vi "Host3.vi"() -> ()   [LabVIEW 2025]
uses:
  <vilib>/Analysis/baseanly.llb/Real Dot Product.vi
  <vilib>/Analysis/baseanly.llb/Real A x B.vi
  <vilib>/Analysis/Matrix/Numeric/Conversions/Matrix To Array - RM.vi
  <vilib>/Utility/error.llb/Error Cluster From Error Code.vi
  <vilib>/rvi/errors/niLvFpgaAdjustHostInterfaceError.vi
  <vilib>/FPGAPlugInAG/Dynamic/niLvFpga_Run_Dynamic.vi
  <vilib>/FPGAPlugInAG/Dynamic/niLvFpga_Close_Dynamic.vi
  <vilib>/rvi/interface/nirviOpenFPGA/nirviOpenFPGA.xnode
  <vilib>/rvi/interface/nirviMethod/nirviMethod.xnode
  <vilib>/rvi/interface/nirviCloseFPGA/nirviCloseFPGA.xnode
  <vilib>/FPGAPlugInAG/Dynamic/niLvFpga_WriteFifo_Dynamic.vi
  <vilib>/rvi/errors/niLvFpgaMergeErrorWithErrorCode.vi
  <vilib>/Analysis/NI_AALBase.lvlib
  <vilib>/Analysis/Matrix/NI_Matrix.lvlib
  <vilib>/FPGAPlugInAG/Dynamic/niLvFpga_ReadFifo_Dynamic.vi
  FPGA Bitfiles/dotplot9033_FPGATarget_Target_CwM8WDNFVFM.lvbitx
  Target.vi
  <vilib>/FPGAPlugInAG/cRIO-9033/niLvFpga_Open_cRIO-9033.vi
  <vilib>/rvi/interface/common/dynamic/niFpgaDynamicAddResources.vi
panel:
  out "FIFO C Output":fxp<+/-,32,16>[](array[numeric])
  out "FIFO A Input":fxp<+/-,32,16>[](array[numeric])
  out "FIFO B Input":fxp<+/-,32,16>[](array[numeric])
  out "X * Y":fxp<+/-,64,32>
  out "elements in B":i32
  out "elements in A":i32
  out "sum of error":dbl
  out "C - FPGA code":fxp<+/-,32,16>[][](array[numeric])
  out "elements in C":i32
  out "C - Real":dbl[][](array[numeric])
  out "B":fxp<+/-,32,16>[][](array[numeric])
  out "A":fxp<+/-,32,16>[][](array[numeric])
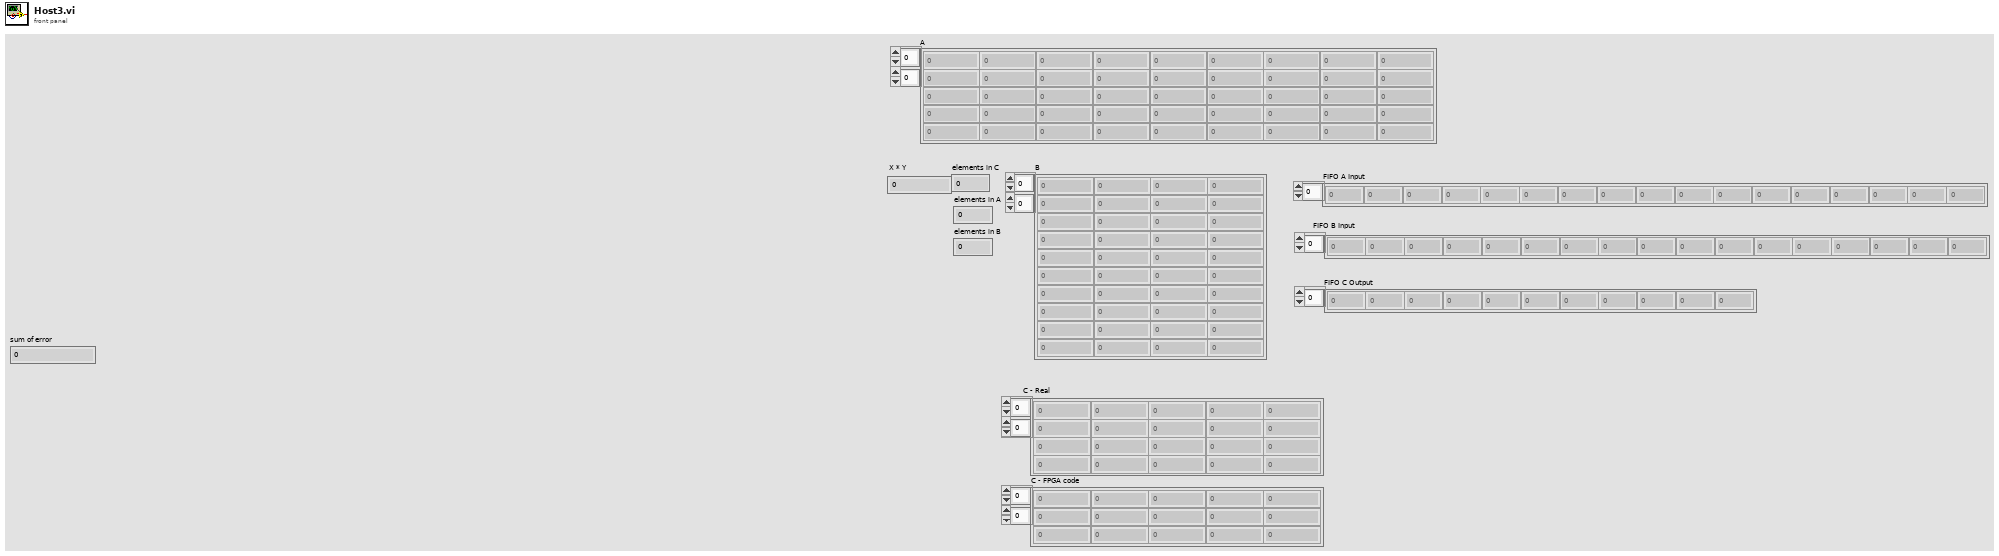
[diagram p1: front panel]
types:
  T1 = typedef "NI_Matrix.lvlib/RealMatrix.ctl" = dbl[][]
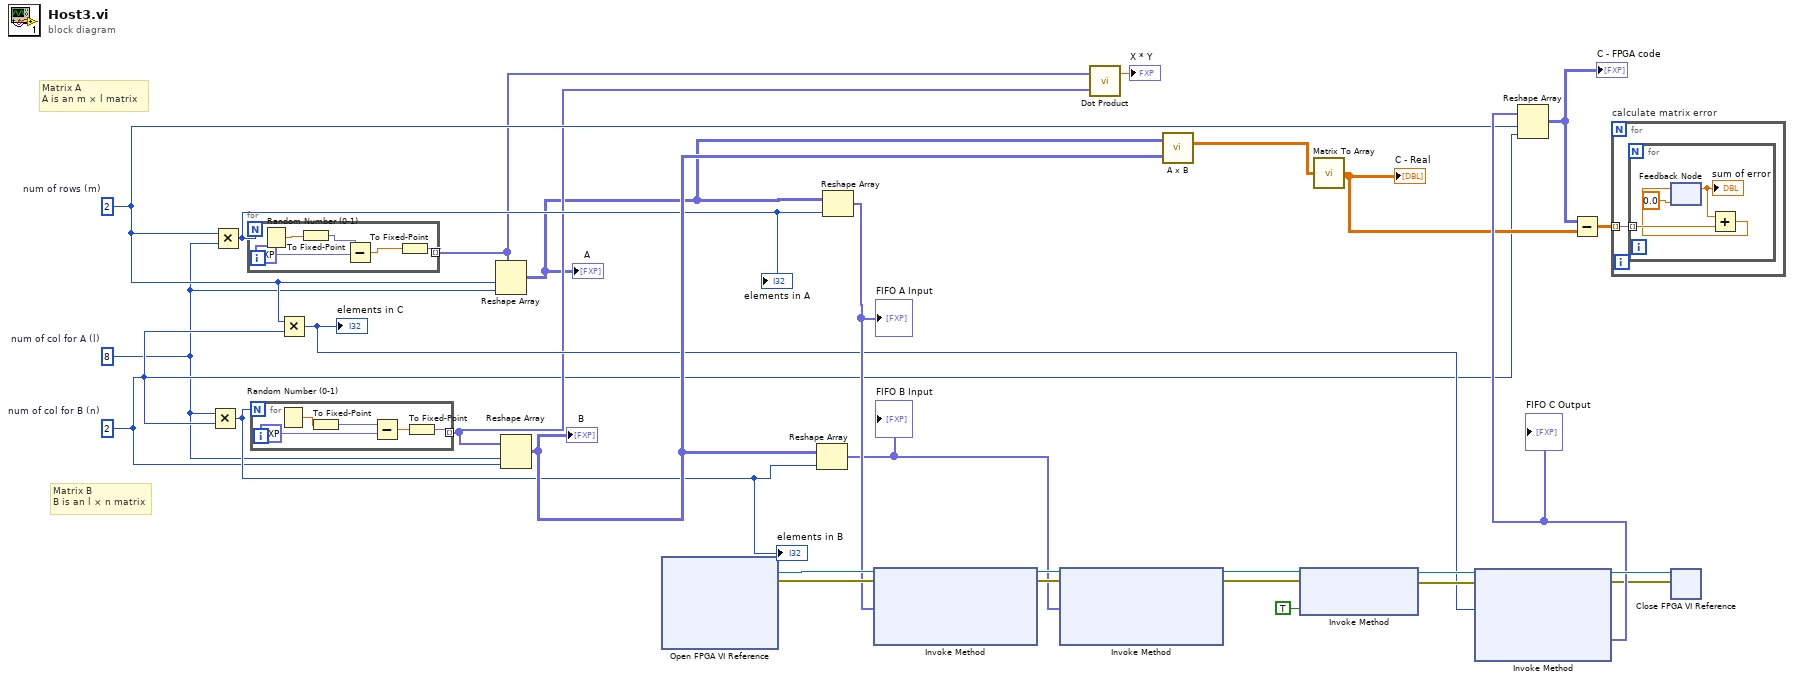
[diagram p0: block diagram]
diagram:
  w3 = 2  # num of col for B (n)
  w2 = 8  # num of col for A (l)
  w12 = 2  # num of rows (m)
  # "Matrix B\nB is an l × n matrix"
  # "Matrix A\nA is an m × l matrix"
  n1 = Multiply(x=w2, y=w3) -> (x*y=w9:i32)
  "elements in B" <- w9
  n2 = Multiply(x=w12, y=w2) -> (x*y=w17:i32)
  "elements in A" <- w17
  n3 = for {
    N: w17 -> [_]
    tunnel: [w32] -> w8 mode=indexing
    n4 = Random Number (0-1)() -> (number: 0 to 1=w33:dbl)
    n5 = To Fixed-Point(number=w33) -> (fixed-point=w30:fxp<+/-,32,16>)  [unwired: 1 in]
    n6 = Subtract(x=w30, y=fxp<+,1,0> 0.5) -> (x-y=w31:sgl)
    n7 = To Fixed-Point(number=w31) -> (fixed-point=w32:fxp<+/-,32,16>)  [unwired: 1 in]
  }
  n8 = for {
    N: w9 -> [_]
    tunnel: [w38] -> w7 mode=indexing
    n9 = Random Number (0-1)() -> (number: 0 to 1=w37:dbl)
    n10 = To Fixed-Point(number=w37) -> (fixed-point=w35:fxp<+/-,32,16>)  [unwired: 1 in]
    n11 = Subtract(x=w35, y=fxp<+,1,0> 0.5) -> (x-y=w36:sgl)
    n12 = To Fixed-Point(number=w36) -> (fixed-point=w38:fxp<+/-,32,16>)  [unwired: 1 in]
  }
  n13 = Multiply(x=w12, y=w3) -> (x*y=w10:i32)
  "elements in C" <- w10
  n14 = Reshape Array(w8, w12, w2) -> (w4:fxp<+/-,32,16>[][])
  "A" <- w4
  n15 = Reshape Array(w7, w2, w3) -> (w19:fxp<+/-,32,16>[][])
  "B" <- w19
  n16 = xnode "Open FPGA VI Reference"() -> ("FPGA VI Reference Out"=w28:refnum<k20>, "error out"=w27:errorcluster)  [unwired: 2 in]
  n17 = Reshape Array(w19, w9) -> (w1:fxp<+/-,32,16>[])
  "FIFO B Input" <- w1
  n18 = Reshape Array(w4, w17) -> (w16:fxp<+/-,32,16>[])
  "FIFO A Input" <- w16
  n19 = xnode "Invoke Method"("FPGA VI Reference In"=w28, "error in"=w27, "Data"=w16) -> ("FPGA VI Reference Out"=w23:refnum<k20>, "error out"=w22:errorcluster)  [unwired: 1 in, 1 out]
  n20 = xnode "Invoke Method"("FPGA VI Reference In"=w23, "error in"=w22, "Data"=w1) -> ("FPGA VI Reference Out"=w21:refnum<k20>, "error out"=w20:errorcluster)  [unwired: 1 in, 1 out]
  n21 = call-poly <vilib>:"Dot Product.vi"("Y Vector"=w7, "X Vector"=w8) -> ("X * Y"=→"X * Y":dbl)  [unwired: 1 out]
  n22 = call-poly <vilib>:"A x B.vi"("B"=w19, "A"=w4) -> ("A x B"=w18:T1)  [unwired: 1 out]
  n23 = xnode "Invoke Method"("FPGA VI Reference In"=w21, "error in"=w20, "Wait Until Done (F)"=TRUE) -> ("FPGA VI Reference Out"=w26:refnum<k20>, "error out"=w25:errorcluster)
  n24 = call-poly <vilib>:"Matrix To Array.vi"("Real Matrix"=w18) -> ("Real 2D Array"=w11:dbl[][])
  "C - Real" <- w11
  n25 = xnode "Invoke Method"("FPGA VI Reference In"=w26, "error in"=w25, "Number of Elements"=w10) -> ("FPGA VI Reference Out"=w24:refnum<k20>, "error out"=w5:errorcluster, "Data"=w13:fxp<+/-,32,16>[])  [unwired: 1 in, 1 out]
  "FIFO C Output" <- w13
  n26 = Reshape Array(w13, w12, w3) -> (w15:fxp<+/-,32,16>[][])
  "C - FPGA code" <- w15
  n27 = Subtract(x=w15, y=w11) -> (x-y=w14:dbl[][])
  n28 = for "calculate matrix error" {
    tunnel: w14 -> [w40] mode=indexing
    n29 = for {
      tunnel: w40 -> [w44] mode=indexing
      n30 = feedback #1(0.0) -> (w42:dbl)
      "sum of error" <- w42
      n31 = Add(x=w42, y=w44) -> (x+y=w43:dbl)
      n32 = feedback-in #1(w43) -> ()
    }
  }
  n33 = xnode "Close FPGA VI Reference"("FPGA VI Reference In"=w24, "error in"=w5) -> ()  [unwired: 1 out]
